vi "update mode in ui.vi"(8 "error in (no error)":errorcluster caption="에러 입력(에러 없음)", 10 "mode":T1, 11 "DW7802 입력":refnum<class "DW7802.lvclass">) -> (0 "error out":errorcluster caption="에러 출력", 3 "DW7802 출력":refnum<class "DW7802.lvclass">)   [LabVIEW 2020, in "DW7802.lvclass"]
uses:
  DW7802.lvclass
  Haptic IC/Controls/(Ctrl)Mode.ctl
  Haptic IC/Haptic IC.lvclass/Haptic IC.ctl
  Haptic IC/Accessors/Read mode ref.vi
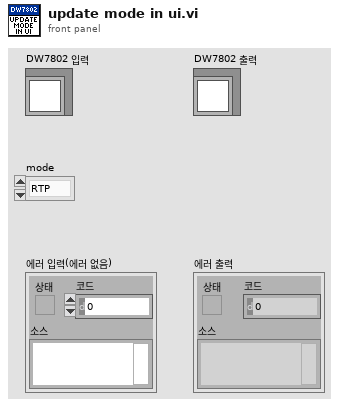
[diagram p1: front panel]
types:
  T1 = typedef "(Ctrl)Mode.ctl" = enum16{"RTP", "Memory"}
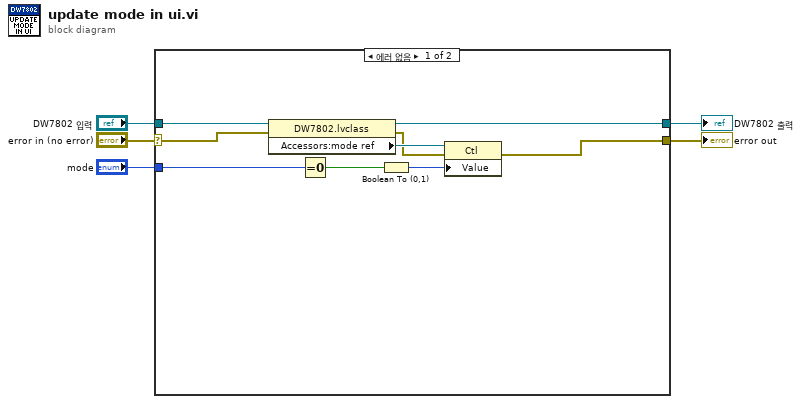
[diagram p0: block diagram]
diagram:
  n1 = case shown="에러 없음" "error in (no error)" {
    selector: "error in (no error)" -> [w14 w15]
    tunnel: "DW7802 입력" -> [w13 w16]
    tunnel: [w9 w15] -> w5
    tunnel: [w12 w16] -> w4
    tunnel: "mode" -> [w8 _]
    frame No Error {
      n2 = property class="DW7802.lvclass"(reference=w13, error in=w14) -> (reference out=w12:refnum<class "DW7802.lvclass">, error out=w10:errorcluster, "Accessors:mode ref"=w11:refnum<vi>)
      n3 = Equal To 0?(x=w8) -> (x = 0?=w7:bool)
      n4 = Boolean To (0,1)(Boolean=w7) -> (0, 1=w6:i16)
      n5 = property class="Ctl"(reference=w11, error in=w10, "Value"=w6) -> (error out=w9:errorcluster)  [unwired: 1 out]
    }
    frame Error {
    }
  }
  "error out" <- w5
  "DW7802 출력" <- w4
